vi "JSON Schema Pretty Print.vi"(5 "String Control":refnum<vi>, 7 "reference":refnum<vi>, 8 "error in (no error)":errorcluster, 11 "<JSON> in":string) -> (0 "error out":errorcluster, 3 "<JSON> out":string)   [LabVIEW 2019, in "JSON-Schema.lvlib"]
uses:
  JSON-Schema.lvlib
  <vilib>/JDP Science/JSONtext/JSONtext.lvlib
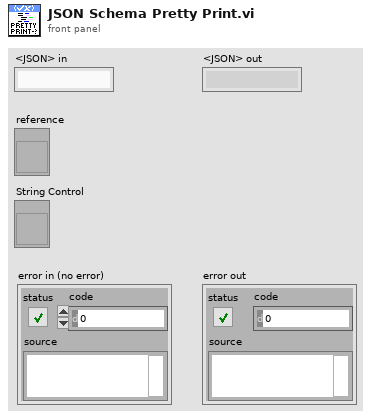
[diagram p1: front panel]
types:
  T1 = enum32{"Bad", "Idle", "Run top level", "Running"}
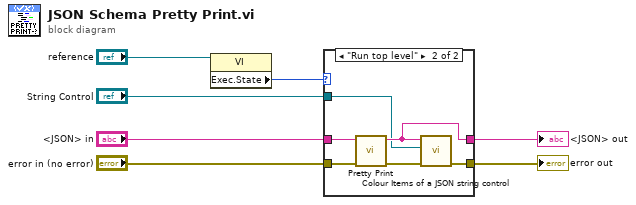
[diagram p0: block diagram]
diagram:
  n1 = property class="VI"(reference="reference") -> ("Exec.State"=w2:T1)  [unwired: 1 in, 2 out]
  n2 = case shown="\"Run top level\"" w2 {
    tunnel: "<JSON> in" -> [w8 w15]
    tunnel: "error in (no error)" -> [w9 w14]
    tunnel: [w9 w12] -> w3
    tunnel: [w8 w11] -> w4
    tunnel: "String Control" -> [_ w10]
    frame Default {
    }
    frame "Run top level" {
      n3 = call <vilib>:"Pretty Print.vi"("error in (no error)"=w14, "JSON"=w15) -> ("error out"=w13:errorcluster, "<JSON>"=w11:string)  [unwired: 7 in, 1 out]
      n4 = call <vilib>:"Colour Items of a JSON string control.vi"("error in (no error)"=w13, "String Control"=w10, "JSON"=w11) -> ("error out"=w12:errorcluster)  [unwired: 8 in]
    }
  }
  "<JSON> out" <- w4
  "error out" <- w3
